vi "g2Cal_Host 160MHz.vi"() -> ()   [LabVIEW 2015]
uses:
  <vilib>/FPGAPlugInAG/USB-7845R/niLvFpga_Open_USB-7845R.vi
  <vilib>/rvi/interface/common/dynamic/niFpgaDynamicAddResources.vi
  <vilib>/Utility/error.llb/Error Cluster From Error Code.vi
  <vilib>/rvi/errors/niLvFpgaAdjustHostInterfaceError.vi
  <vilib>/rvi/interface/nirviOpenFPGA/nirviOpenFPGA.xnode
  FPGA Bitfiles/UntitledProject1_FPGATarget_g2Calsim160MHz_YGyXm5ymhbo.lvbitx
  g2Cal sim 160MHz.vi
  <vilib>/rvi/interface/nirviReadWriteControl/nirviReadWriteControl.xnode
  <vilib>/rvi/interface/nirviMethod/nirviMethod.xnode
  <vilib>/FPGAPlugInAG/Dynamic/niLvFpga_ReadFifo_Dynamic.vi
  <vilib>/rvi/errors/niLvFpgaMergeErrorWithErrorCode.vi
  NiFpgaLv.dll
  <vilib>/rvi/interface/Simulation/niFpgaSimulationCallBeginRW.vi
panel:
  out "ms 타이머 값":u32
  out "Data pulling":bool
  out "남아있는 원소":u32
  out "배열":u32[](array[numeric])
  in  "Frequency (MHz)":fxp<+,32,4>=1.0
  out "웨이브폼 그래프":u32[](graph)
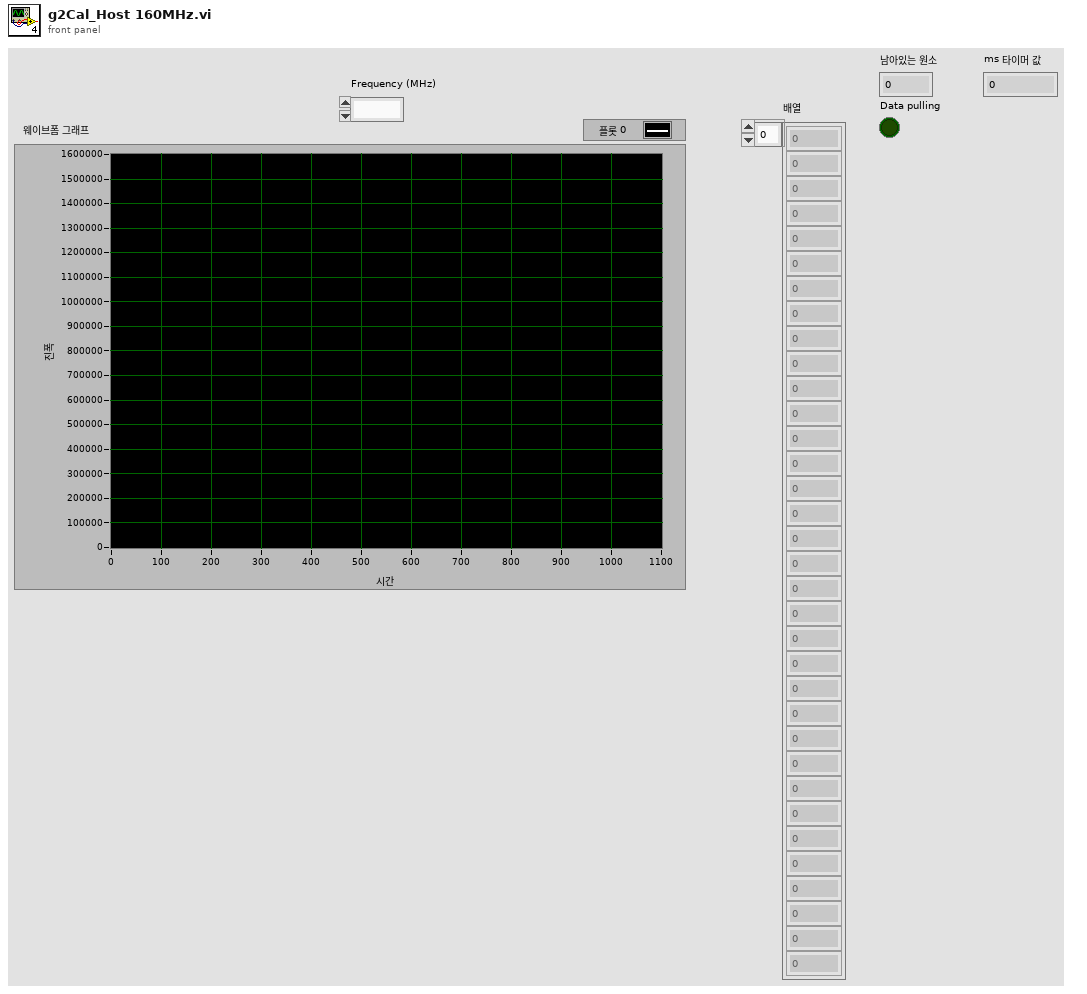
[diagram p1: front panel]
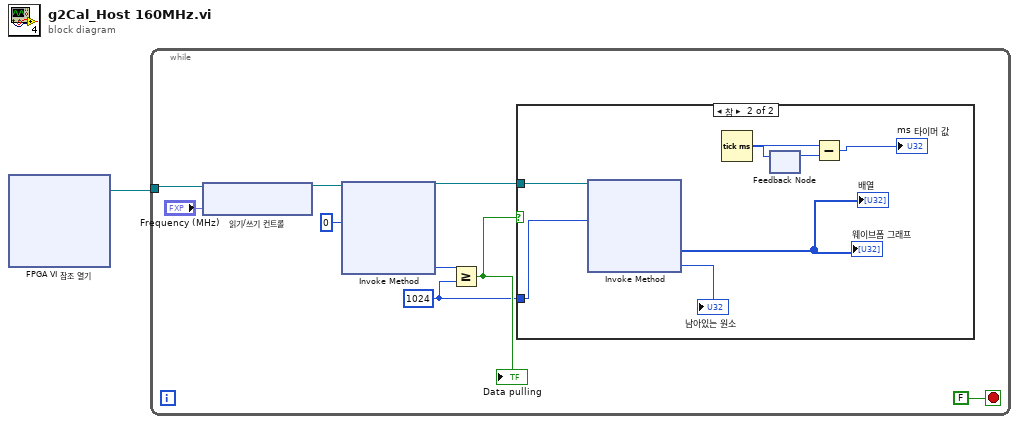
[diagram p0: block diagram]
diagram:
  n1 = xnode "FPGA VI 참조 열기"() -> ("FPGA VI 참조 출력"=w1:refnum<k20>)  [unwired: 2 in, 1 out]
  n2 = while {
    tunnel: w1 -> [w5]
    stop <- FALSE stop-if-true
    w2 = u32 1024 ("y")
    n3 = xnode "읽기/쓰기 컨트롤"("FPGA VI 참조 입력"=w5, "Frequency (MHz)"="Frequency (MHz)") -> ("FPGA VI 참조 출력"=w4:refnum<k20>)  [unwired: 1 in, 1 out]
    n4 = xnode "Invoke Method"("FPGA VI 참조 입력"=w4, "원소의 개수"=u32 0) -> ("FPGA VI 참조 출력"=w7:refnum<k20>, "남아있는 원소"=w9:u32)  [unwired: 2 in, 2 out]
    n5 = Greater Or Equal?(x=w9, y=w2) -> (x >= y?=w8:bool)
    "Data pulling" <- w8
    n6 = case shown="참" w8 {
      tunnel: w7 -> [_ w17]
      tunnel: w2 -> [_ w14]
      frame False {
      }
      frame True {
        n7 = xnode "Invoke Method"("FPGA VI 참조 입력"=w17, "원소의 개수"=w14) -> ("데이터"=→"웨이브폼 그래프" →"배열":u32[], "남아있는 원소"=→"남아있는 원소":u32)  [unwired: 2 in, 2 out]
        n8 = Tick Count (ms)() -> (millisecond timer value=w12:u32)
        n9 = feedback #1 ("피드백 노드")() -> (w13:u32)  [unwired: 1 in]
        n10 = feedback-in #1(w12) -> ()
        n11 = Subtract(x=w12, y=w13) -> (x-y=→"ms 타이머 값":u32)
      }
    }
  }
